vi "PE Set Wavelength.vi"(8 "error in (no error)":errorcluster, 10 "wavelength":dbl, 11 "peHandle":u64) -> (0 "error out":errorcluster)   [LabVIEW 2015, in "PE_Filter_SDK.lvlib"]
doc: "PEFILTERSDK_API PE_STATUS PE_SetWavelength(PE_HANDLE peHandle, double wavelength);"
uses:
  Documents/test/SDK 1.2.4 Installer/SDK 1.2.4 Installer/examples/Labview/win64/PE_Filter_SDK/PE_Filter_SDK.lvlib
  Documents/test/SDK 1.2.4 Installer/SDK 1.2.4 Installer/win64/PE_Filter_SDK.dll
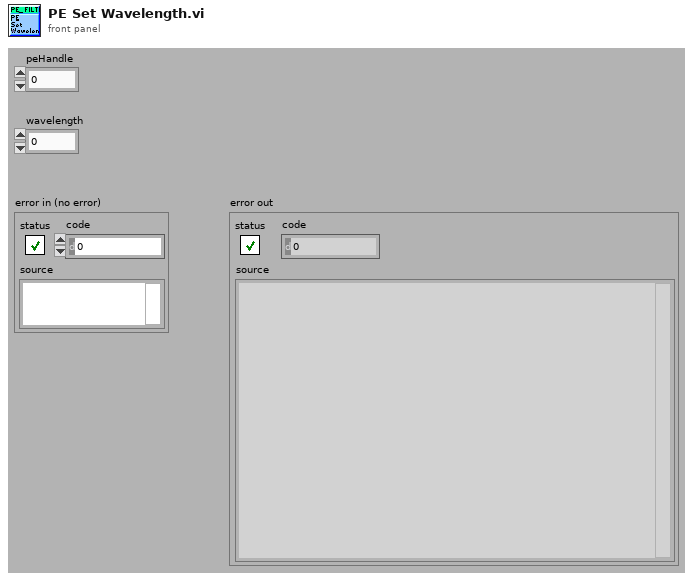
[diagram p1: front panel]
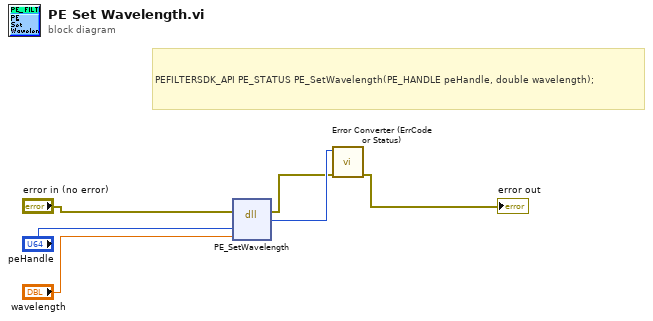
[diagram p0: block diagram]
diagram:
  # "PEFILTERSDK_API PE_STATUS PE_SetWavelength(PE_HANDLE peHandle, double wavelength);"
  n1 = dll-call lib="C:/Users/localAdmin/Documents/test/SDK 1.2.4 Installer/SDK 1.2.4 Installer/win64/PE_Filter_SDK.dll" fn="PE_SetWavelength"(error in="error in (no error)", "peHandle"="peHandle", "wavelength"="wavelength") -> (error out=w2:errorcluster, "return type"=w3:i32)  [unwired: 4 in, 1 out]
  n2 = call "Error Converter (ErrCode or Status).vi"("error in (no error)"=w2, "error code"=w3) -> ("error out"=→"error out":errorcluster)  [unwired: 9 in]
